vi "_QMH_Enqueue.vi"(6 "timeout in ms (-1)":i32=-1, 8 "error in (no error)":errorcluster, 9 "Data":variant, 10 "Msg":string, 11 "QMH in":refnum<class "QMH.lvclass">) -> (0 "error out":errorcluster, 3 "QMH out":refnum<class "QMH.lvclass">)   [LabVIEW 2018, in "QMH.lvclass"]
uses:
  QMH.lvclass
  QMH.lvclass/QMH.ctl
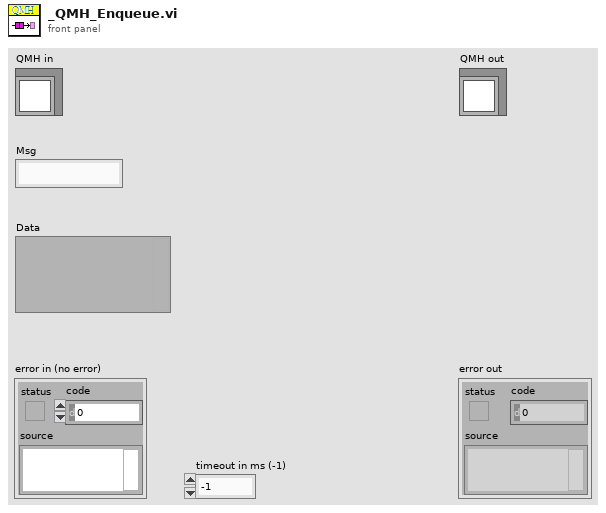
[diagram p1: front panel]
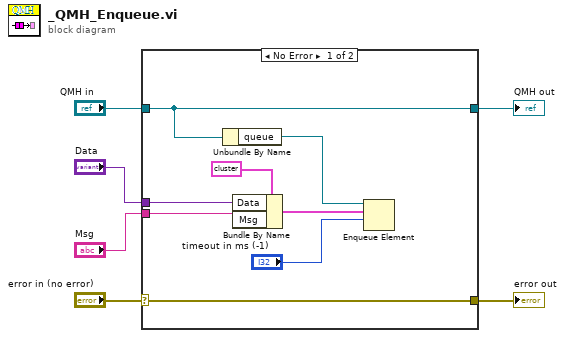
[diagram p0: block diagram]
diagram:
  n1 = case shown="No Error" "error in (no error)" {
    selector: "error in (no error)" -> [w14 w16]
    tunnel: [w14 w16] -> w5
    tunnel: [w13 w15] -> w3
    tunnel: "QMH in" -> [w13 w15]
    tunnel: "Data" -> [w8 _]
    tunnel: "Msg" -> [w7 _]
    frame No Error {
      n2 = Unbundle By Name(w13) -> ("queue"=w12:refnum<queue>)
      n3 = Bundle By Name(cluster=cluster{"Data":variant, "Msg":string} {"Data"=variant, "Msg"=""} ("QM in"), "Data"=w8, "Msg"=w7) -> (w9:cluster{"Data":variant, "Msg":string})
      n4 = Enqueue Element(queue=w12, element=w9, timeout in ms (-1)="timeout in ms (-1)") -> ()  [unwired: 1 in, 3 out]
    }
    frame Error {
    }
  }
  "error out" <- w5
  "QMH out" <- w3
